vi "Sam_AskToSave.vi"(10 "Data":waveform(dbl)[][](array[waveform]), 11 "Names":string[](array[string])) -> ()   [LabVIEW 2022 SP3]
panel:
  in  "Play":bool
  in  "Files":u16(ring) items=["Test 2 H", "Test 3 V", "Test 5 V"]
  in  "Save":bool
  out "Hammer":waveform(dbl)(graph)
  out "Microphone":waveform(dbl)(graph)
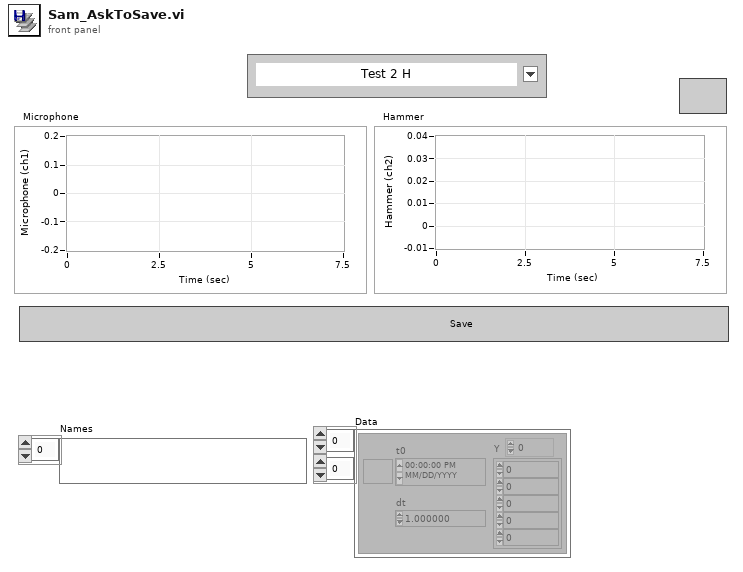
[diagram p1: front panel]
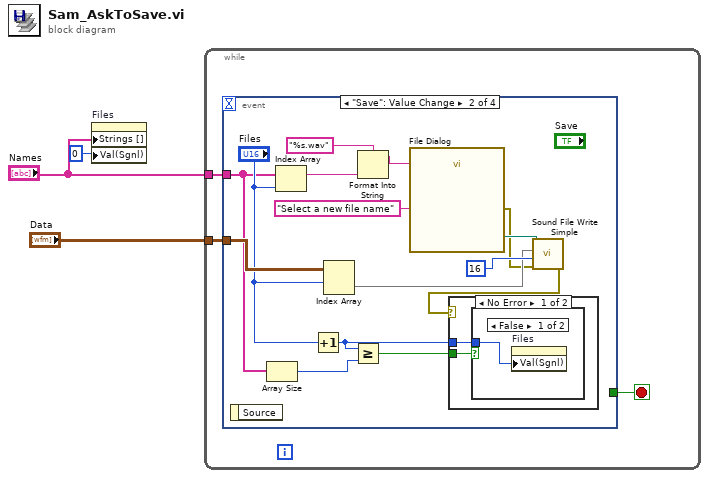
[diagram p0: block diagram]
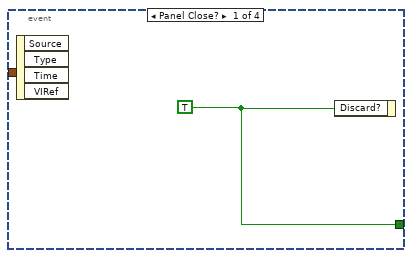
[diagram p2: hidden frame]
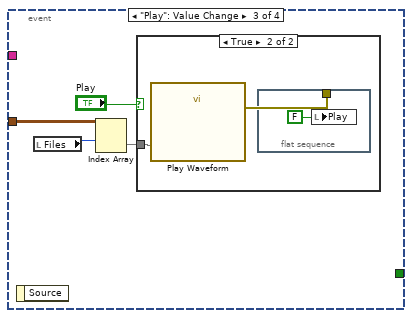
[diagram p5: hidden frame]
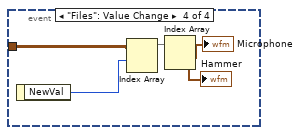
[diagram p7: hidden frame]
diagram:
  n1 = property on="Files" class="Ring (strict)"("Strings []"="Names", "Val(Sgnl)"=u16 0 ("Value (Signaling)")) -> ()  [unwired: 2 in, 2 out]
  n2 = while {
    tunnel: "Data" -> [w5]
    tunnel: "Names" -> [w4]
    stop <- w6 stop-if-true
    n3 = event shown="[1] \"Save\": Value Change" {
      selector: _ -> [_ _ _ _]
      dyn-events: _ -> [_ _ _ _]
      timeout: _ -> [_ _ _ _]
      tunnel: [w7 _ _ _] -> w6
      tunnel: w5 -> [_ w18 w29 w37]
      tunnel: w4 -> [_ w12 _ _]
      event Panel Close? {
        w7 = TRUE ("Discard?")
        n4 = event-data() -> ()  [unwired: 1 in, 4 out]
        n5 = event-data("Discard?"=w7) -> ()  [unwired: 1 in, 1 out]
      }
      event "Save": Value Change {
        n6 = event-data() -> ()  [unwired: 1 in, 1 out]
        n7 = Array Size(array=w12) -> (size(s)=w11:i32)
        n8 = Index Array(array=w12, index="Files") -> (element=w16:string)
        n9 = Increment(x="Files") -> (x+1=w9:u16)
        n10 = Index Array(array=w18, index (row)="Files") -> (element=w19:waveform(dbl)[])  [unwired: 1 in]
        n11 = Greater Or Equal?(x=w9, y=w11) -> (x >= y?=w10:bool)
        n12 = Format Into String(format string="%s.wav" ("default name"), w16) -> (resulting string=w15:string)  [unwired: 2 in, 1 out]
        n13 = call "File Dialog"("prompt"="Select a new file name", "default name"=w15) -> ("selected path"=w20:path, "error out"=w14:errorcluster)  [unwired: 10 in, 2 out]
        n14 = call <vilib>:"Sound File Write Simple.vi"("error in (no error)"=w14, "bits per sample"=16, "data"=w19, "path"=w20) -> ("error out"=w8:errorcluster)  [unwired: 6 in, 1 out]
        n15 = case shown="No Error" w8 {
          tunnel: w10 -> [w24 _]
          tunnel: w9 -> [w23 _]
          frame No Error {
            n16 = case shown="False" w24 {
              tunnel: w23 -> [w25 _]
              frame False {
                n17 = property on="Files" class="Ring (strict)"("Val(Sgnl)"=w25) -> ()  [unwired: 2 in, 2 out]
              }
              frame True {
              }
            }
          }
          frame Error {
          }
        }
      }
      event "Play": Value Change {
        n18 = event-data() -> ()  [unwired: 1 in, 1 out]
        n19 = local read "Files"() -> (w28:u16)
        n20 = Index Array(array=w29, index (row)=w28) -> (element=w27:waveform(dbl)[])  [unwired: 1 in]
        n21 = case shown="True" "Play" {
          tunnel: w27 -> [_ w31]
          frame False {
          }
          frame True {
            n22 = call "Play Waveform"("Data"=w31) -> ("error out"=w30:errorcluster)  [unwired: 18 in]
            n23 = flat-sequence {
              tunnel: w30 -> [_]
              frame #0 {
                n24 = local write "Play"(FALSE) -> ()
              }
            }
          }
        }
      }
      event "Files": Value Change {
        n25 = event-data() -> ("NewVal"=w36:u16)  [unwired: 1 in]
        n26 = Index Array(array=w37, index (row)=w36) -> (element=w35:waveform(dbl)[])  [unwired: 1 in]
        n27 = Index Array(array=w35) -> (element #1=→"Microphone":waveform(dbl), element #2=→"Hammer":waveform(dbl))  [unwired: 2 in]
      }
    }
  }
